vi "stepper controller -- IMS.vi"(7 "stepper motor action":T2, 8 "set":dbl format="%#_13g", 9 "stepper motor state":T1) -> (1 "stepper motor state OUT":T1)   [LabVIEW 2018]
uses:
  stepper motor state.ctl
  stepper motor action.ctl
  internal stepper state.ctl
panel:
  in  "VISA session":refnum<visa-resource-name>="GPIB0::25::INSTR"
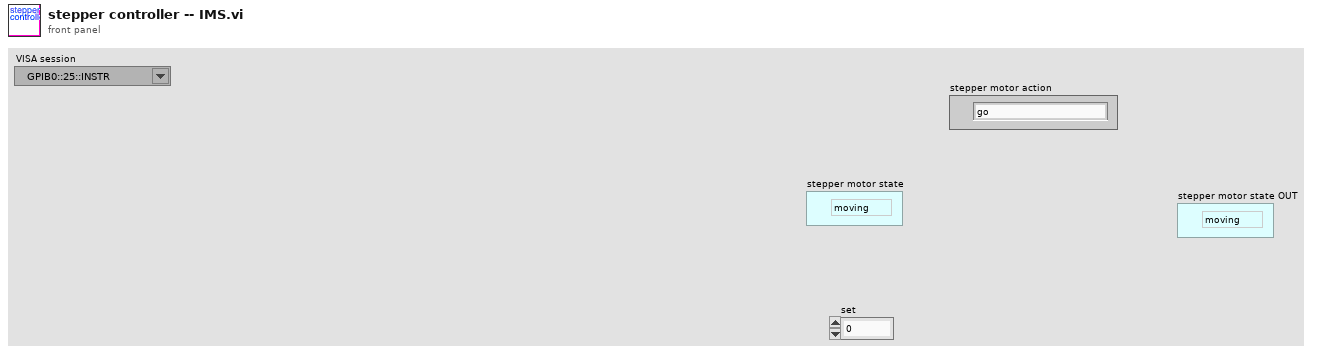
[diagram p1: front panel]
types:
  T1 = typedef "stepper motor state.ctl" = enum16{"moving", "stopped"}
  T2 = typedef "stepper motor action.ctl" = enum16{"go", "stop", "check", "init", "sync", "set"}
  T3 = cluster{"initialized?":bool, "VISA session":refnum<visa-resource-name>}
  T4 = typedef "internal stepper state.ctl" = cluster{"initialized?":bool, "VISA address":refnum<visa-resource-name>}
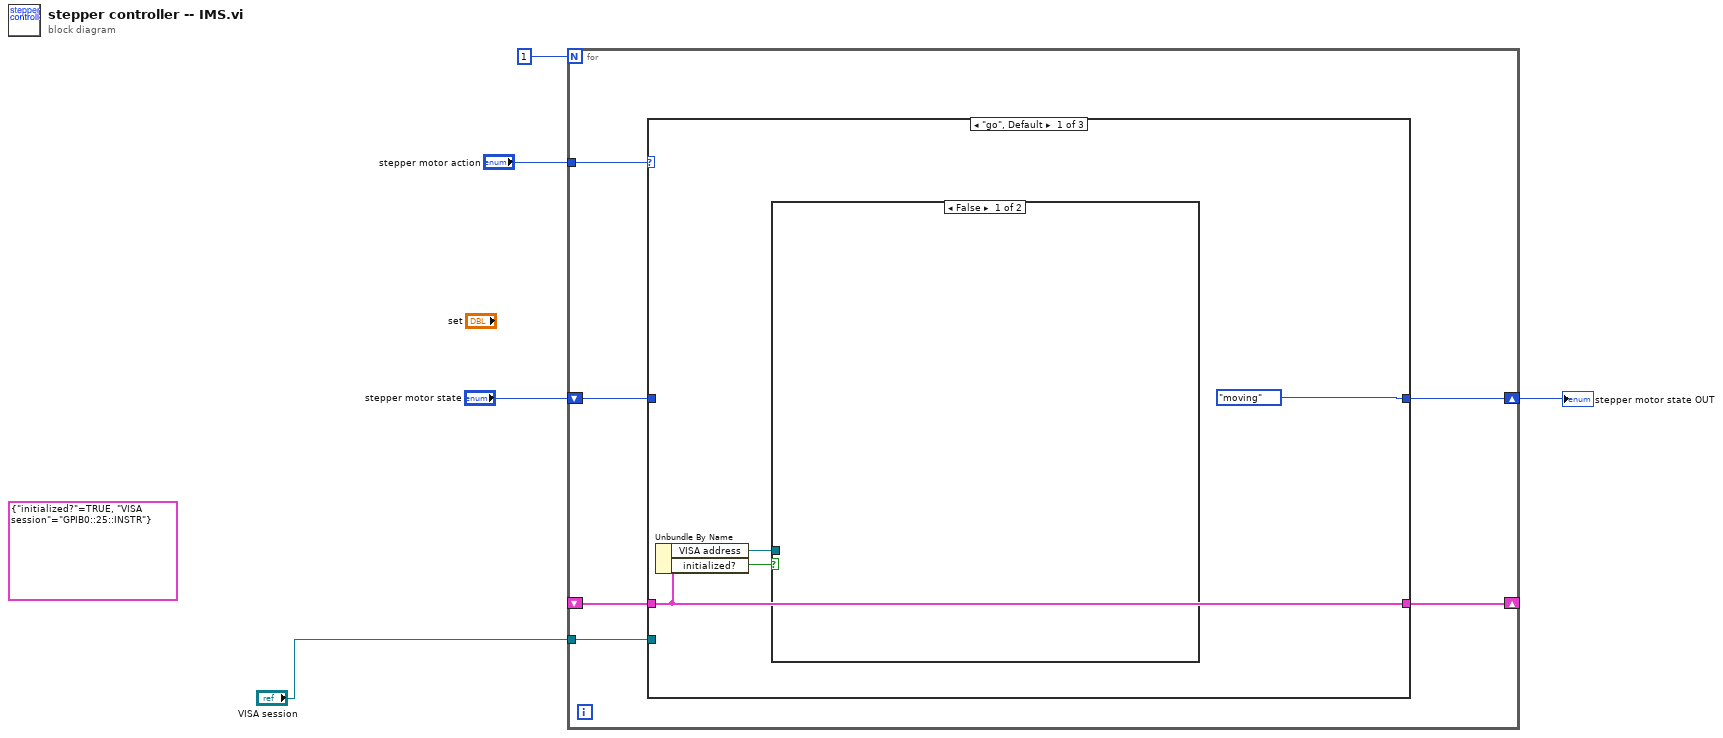
[diagram p0: block diagram]
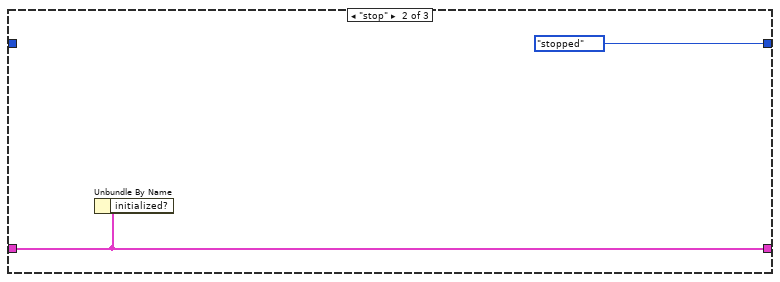
[diagram p3: hidden frame]
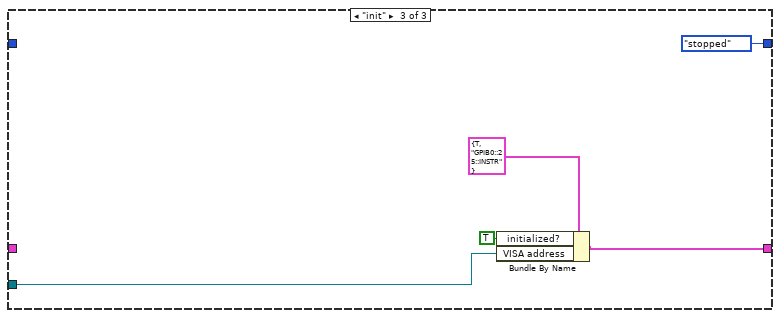
[diagram p4: hidden frame]
diagram:
  (unwired) T3 {"initialized?"=TRUE, "VISA session"="GPIB0::25::INSTR"}
  n1 = for {
    N: 1 -> [_]
    tunnel: "stepper motor action" -> [w11]
    shift-right: [w10] -> w4
    shift-left: "stepper motor state" -> [w9]
    shift-right: [w8] -> _
    shift-left: _ -> [w7]
    tunnel: "VISA session" -> [w6]
    n2 = case shown="\"go\", Default" w11 {
      tunnel: w9 -> [_ _ _]
      tunnel: [stepper_motor_state."moving" ("stepper motor state") stepper_motor_state."stopped" ("stepper motor state") stepper_motor_state."stopped" ("stepper motor state")] -> w10
      tunnel: [w14 w16 w21] -> w8
      tunnel: w7 -> [w14 w16 _]
      tunnel: w6 -> [_ _ w18]
      frame "go", Default {
        n3 = Unbundle By Name(w14) -> ("VISA address"=w12:refnum<visa-resource-name>, "initialized?"=w13:bool)
        n4 = case shown="False" w13 {
          tunnel: w12 -> [_ _]
          frame False {
          }
          frame True {
          }
        }
      }
      frame "stop" {
        n5 = Unbundle By Name(w16) -> ()  [unwired: 1 out]
      }
      frame "init" {
        n6 = Bundle By Name(cluster=T4 {"initialized?"=TRUE, "VISA address"="GPIB0::25::INSTR"} ("internal stepper state"), "initialized?"=TRUE, "VISA address"=w18) -> (w21:T4)
      }
    }
  }
  "stepper motor state OUT" <- w4
